vi "SaveTabFocus.vi"(8 "error in (no error)":errorcluster, 11 "GuiderSetup in":refnum<class "GuiderSetup.lvclass">) -> (0 "error out":errorcluster, 3 "GuiderSetup out":refnum<class "GuiderSetup.lvclass">)   [LabVIEW 2018, in "GuiderSetup.lvclass"]
uses:
  GuiderSetup.lvclass
  C:/Users/devstaff/sparc4/s4gui/Versao ZeroMQ REQ-REP/SPARC4_GUI -v1.0.0 - 20241216/S4GUI/S4GUI.lvclass
  S4GUI/S4GUI.lvclass/S4GUI.ctl
  <vilib>/Utility/config.llb/Write Key (Double).vi
  Instrument/Instrument.lvclass
  S4GUI/S4GUI.lvclass
  <vilib>/Utility/config.llb/NI_LVConfig.lvlib
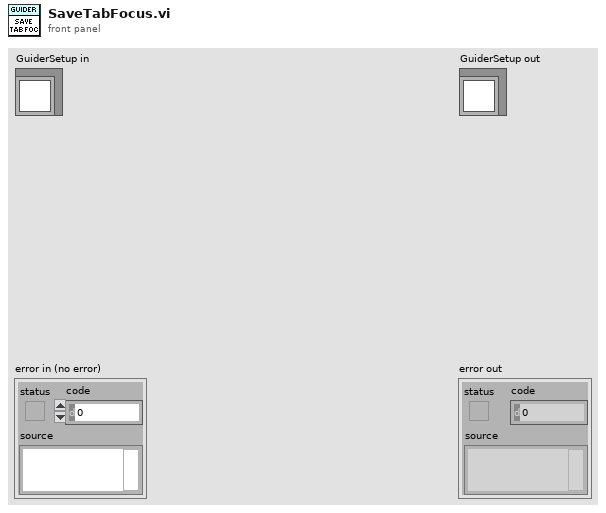
[diagram p1: front panel]
types:
  T1 = cluster{"Photometric":dbl, " Polarimetry":dbl, "Polarimetry \nEfficiency":dbl, "Instrumental polarization":dbl}
  T2 = typedef "NI_LVConfig.lvlib/Config Data RefNum.ctl" = refnum<k1>
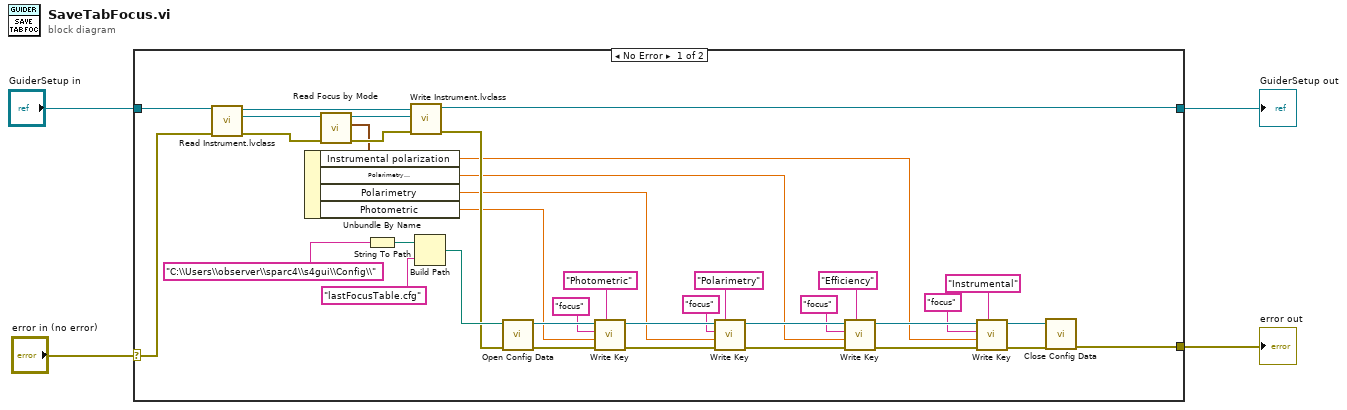
[diagram p0: block diagram]
diagram:
  n1 = case shown="No Error" "error in (no error)" {
    selector: "error in (no error)" -> [w13 w43]
    tunnel: [w6 w43] -> w3
    tunnel: [w37 w42] -> w1
    tunnel: "GuiderSetup in" -> [w38 w42]
    frame No Error {
      n2 = call "Read Instrument.lvclass.vi"("error in (no error)"=w13, "S4ACS_GUI in"=w38) -> ("error out"=w36:errorcluster, "Instrument.lvclass"=w40:refnum<class "Instrument.lvclass">, "S4ACS_GUI out"=w41:refnum<class "GuiderSetup.lvclass">)  [unwired: 7 in]
      n3 = call-dynamic "Read Focus by Mode.vi"("error in (no error)"=w36, "Instrument in"=w40) -> ("error out"=w35:errorcluster, "Focus by Mode"=w11:T1, "Instrument out"=w39:refnum<class "Instrument.lvclass">)  [unwired: 7 in]
      n4 = Unbundle By Name(w11) -> ("Instrumental polarization"=w9:dbl, "Polarimetry \nEfficiency"=w8:dbl, "Polarimetry"=w7:dbl, "Photometric"=w10:dbl)
      n5 = String To Path(string="C:\\Users\\observer\\sparc4\\s4gui\\Config\\") -> (path=w26:path)
      n6 = call "Write Instrument.lvclass.vi"("error in (no error)"=w35, "Instrument.lvclass"=w39, "S4ACS_GUI in"=w41) -> ("error out"=w12:errorcluster, "S4ACS_GUI out"=w37:refnum<class "GuiderSetup.lvclass">)  [unwired: 7 in]
      n7 = Build Path(base path=w26, name or relative path="lastFocusTable.cfg") -> (appended path=w23:path)
      n8 = call <vilib>:"Open Config Data.vi"("error in (no error)"=w12, "configuration file path"=w23) -> ("error out"=w25:errorcluster, "refnum"=w24:T2)  [unwired: 7 in, 1 out]
      n9 = call-poly <vilib>:"Write Key.vi"("section"="Photometric" ("key"), "error in (no error)"=w25, "value"=w10, "key"="focus", "refnum"=w24) -> ("error out"=w29:errorcluster, "refnum out"=w27:T2)  [unwired: 4 in, 1 out]
      n10 = call-poly <vilib>:"Write Key.vi"("section"="Polarimetry" ("key"), "error in (no error)"=w29, "value"=w7, "key"="focus", "refnum"=w27) -> ("error out"=w30:errorcluster, "refnum out"=w28:T2)  [unwired: 4 in, 1 out]
      n11 = call-poly <vilib>:"Write Key.vi"("section"="Efficiency" ("key"), "error in (no error)"=w30, "value"=w8, "key"="focus", "refnum"=w28) -> ("error out"=w33:errorcluster, "refnum out"=w31:T2)  [unwired: 4 in, 1 out]
      n12 = call-poly <vilib>:"Write Key.vi"("section"="Instrumental" ("key"), "error in (no error)"=w33, "value"=w9, "key"="focus", "refnum"=w31) -> ("error out"=w34:errorcluster, "refnum out"=w32:T2)  [unwired: 4 in, 1 out]
      n13 = call <vilib>:"Close Config Data.vi"("error in (no error)"=w34, "refnum"=w32) -> ("error out"=w6:errorcluster)  [unwired: 8 in, 1 out]
    }
    frame Error {
    }
  }
  "error out" <- w3
  "GuiderSetup out" <- w1
